vi "Clear Hardware.vi"(2 "error in (no error)":errorcluster, 3 "NI Card in":refnum<class "NI Card.lvclass">) -> (0 "error out":errorcluster, 1 "NI Card out":refnum<class "NI Card.lvclass">)   [LabVIEW 2013, in "NI Card.lvclass"]
uses:
  NI Card.lvclass
  NI Card.lvclass/NI Card.ctl
  <vilib>/DAQmx/read.llb/DAQmx Read (Analog 1D DBL NChan 1Samp).vi
  <vilib>/DAQmx/read.llb/DAQmx Read (Analog 1D Wfm NChan NSamp).vi
  <vilib>/DAQmx/write.llb/DAQmx Write (Analog 1D DBL NChan 1Samp).vi
  <vilib>/DAQmx/miscellaneous.llb/DAQmx Fill In Error Info.vi
  <vilib>/Waveform/WDTOps.llb/WDT Append Waveforms DBL.vi
  <resource>/objmgr/daqmx.rc
panel:
  out "AI Data":cluster{dbl[], "Y":dbl[], "String":string}[](array[cluster])
  out "data":waveform(dbl)[](graph)
  out "First Data Point":dbl[](array[numeric]) format="%0.2f"
  out "Number of points read":i32[](array[numeric])
  in  "Set to zero":bool
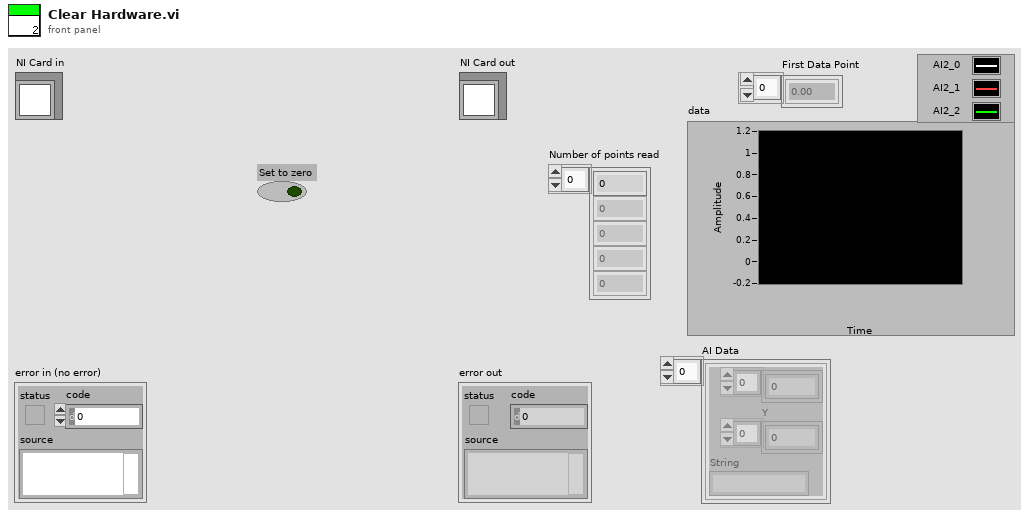
[diagram p1: front panel]
types:
  T1 = cluster{"DAQmx Global Channel":refnum<k21>, "String":string}[]
  T2 = typedef "NI Card.lvclass/AI_Data.ctl" = cluster{"t":dbl[], "y":dbl[], "Channel Name":string}
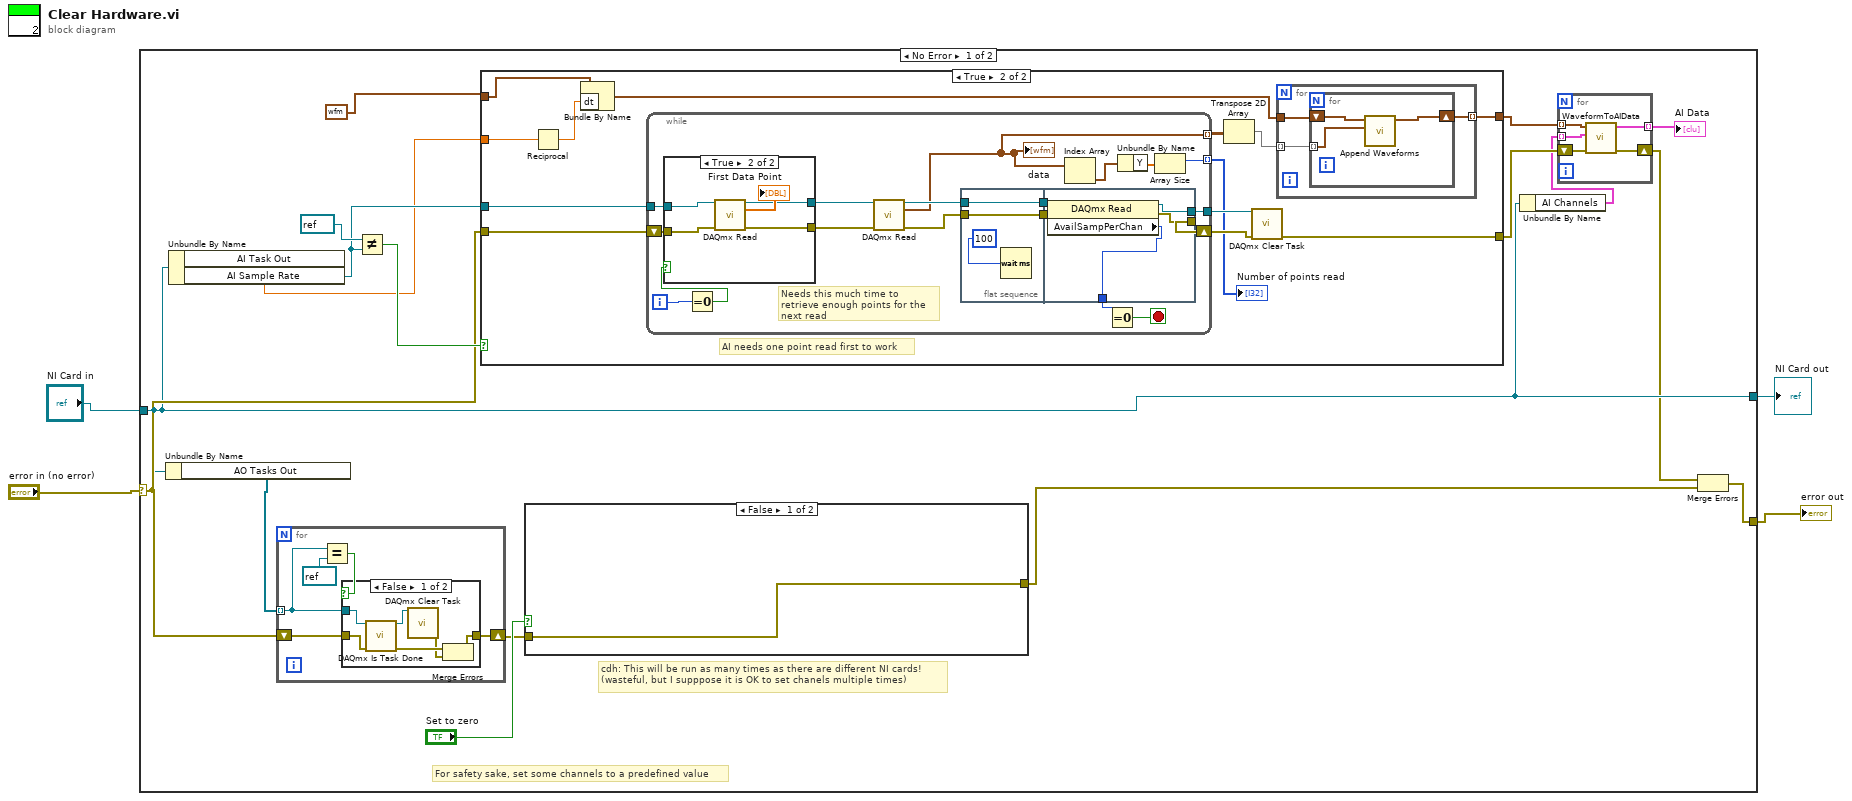
[diagram p0: block diagram]
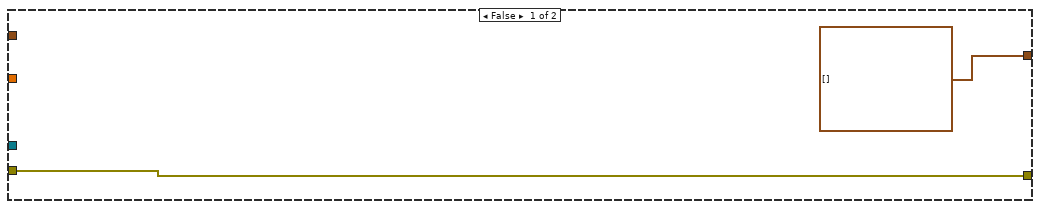
[diagram p2: hidden frame]
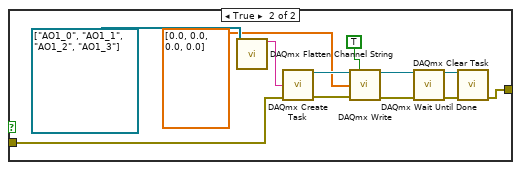
[diagram p5: hidden frame]
diagram:
  n1 = case shown="No Error" "error in (no error)" {
    selector: "error in (no error)" -> [w16 w106]
    tunnel: [w10 w107] -> w1
    tunnel: "NI Card in" -> [w10 w107]
    tunnel: [w6 w106] -> w2
    frame No Error {
      # "cdh: This will be run as many times as there are different NI cards!\n(wasteful, but I supppose it is OK to set chanels multiple times)"
      # "For safety sake, set some channels to a predefined value"
      n2 = Unbundle By Name(w10) -> ("AO Tasks Out"=w21:refnum<k21>[])
      n3 = Unbundle By Name(w10) -> ("AI Task Out"=w15:refnum<k21>, "AI Sample Rate"=w14:dbl)
      n4 = for {
        shift-right: [w82] -> w19
        shift-left: w16 -> [w85]
        tunnel: w21 -> [w81] mode=indexing
        n5 = Equal?(x=w81, y=refnum<k21> refnum ("Name")) -> (x = y?=w83:bool)
        n6 = case shown="False" w83 {
          tunnel: w85 -> [w89 w92]
          tunnel: [w86 w92] -> w82
          tunnel: w81 -> [w91 _]
          frame False {
            n7 = call <vilib>:"DAQmx Is Task Done.vi"("task/channels in"=w91, "error in"=w89) -> ("task out"=w90:refnum<k21>, "error out"=w88:errorcluster)  [unwired: 11 in, 1 out]
            n8 = call <vilib>:"DAQmx Clear Task.vi"("task in"=w90) -> ("error out"=w87:errorcluster)  [unwired: 1 in, 13 out]
            n9 = Merge Errors(w88, w87) -> (w86:errorcluster)
          }
          frame True {
          }
        }
      }
      n10 = Not Equal?(x=refnum<k21> refnum ("task out"), y=w15) -> (x != y?=w17:bool)
      n11 = case shown="True" w17 {
        tunnel: w15 -> [_ w38]
        tunnel: w16 -> [w27 w37]
        tunnel: [w27 w36] -> w11
        tunnel: [waveform(dbl)[] [] w33] -> w12
        tunnel: waveform(dbl) {"t0"=timestamp(0 s since 1904-01-01), "dt"=0.001, "Y"=[]} ("Waveform") -> [_ w31]
        tunnel: w14 -> [_ w29]
        frame False {
        }
        frame True {
          # "AI needs one point read first to work"
          n12 = Reciprocal(x=w29) -> (1/x=w30:dbl)
          n13 = Bundle By Name(cluster=w31, "dt"=w30) -> (w32:waveform(dbl))
          n14 = while {
            tunnel: w38 -> [w64]
            tunnel: [w58] -> w39 mode=indexing
            tunnel: [w54] -> w40
            tunnel: [w48] -> w35 mode=indexing
            shift-right: [w53] -> w41
            shift-left: w37 -> [w63]
            i -> [w51]
            stop <- w57 stop-if-true
            # "Needs this much time to retrieve enough points for the next read"
            n15 = Equal To 0?(x=w51) -> (x = 0?=w50:bool)
            n16 = case shown="True" w50 {
              tunnel: w64 -> [w67 w72]
              tunnel: w63 -> [w66 w71]
              tunnel: [w67 w69] -> w62
              tunnel: [w66 w68] -> w61
              frame False {
              }
              frame True {
                n17 = call-poly <vilib>:"DAQmx Read.vi"("task/channels in"=w72, "error in"=w71) -> ("task out"=w69:refnum<k21>, "data"=→"First Data Point":dbl[], "error out"=w68:errorcluster)  [unwired: 11 out]
              }
            }
            n18 = call-poly <vilib>:"DAQmx Read.vi"("task/channels in"=w62, "error in"=w61) -> ("task out"=w60:refnum<k21>, "data"=w48:waveform(dbl)[], "error out"=w59:errorcluster)  [unwired: 1 in, 10 out]
            "data" <- w48
            n19 = flat-sequence {
              tunnel: w60 -> [w74]
              tunnel: w59 -> [w73]
              tunnel: [w74] -> w56
              tunnel: [w73] -> w55
              tunnel: w56 -> [w80]
              tunnel: w55 -> [w79]
              tunnel: [w78] -> w54
              tunnel: [w77] -> w53
              tunnel: [w76] -> w52
              frame #0 {
                n20 = Wait (ms)(milliseconds to wait=u32 100) -> ()  [unwired: 1 out]
              }
              frame #1 {
                n21 = property class="DAQmx Read"(reference=w80, error in=w79) -> (reference out=w78:refnum<k21>, error out=w77:errorcluster, "AvailSampPerChan"=w76:u32)
              }
            }
            n22 = Index Array(array=w48) -> (element=w49:waveform(dbl))  [unwired: 1 in]
            n23 = Equal To 0?(x=w52) -> (x = 0?=w57:bool)
            n24 = Unbundle By Name(w49) -> ("Y"=w65:dbl[])
            n25 = Array Size(array=w65) -> (size(s)=w58:i32)
          }
          "Number of points read" <- w39
          n26 = Transpose 2D Array(2D array=w35) -> (transposed array=w34:waveform(dbl)[][])
          n27 = call <vilib>:"DAQmx Clear Task.vi"("task in"=w40, "error in"=w41) -> ("error out"=w36:errorcluster)  [unwired: 13 out]
          n28 = for {
            tunnel: w34 -> [w42] mode=indexing
            tunnel: [w43] -> w33 mode=indexing
            tunnel: w32 -> [w44]
            n29 = for {
              tunnel: w42 -> [w45] mode=indexing
              shift-right: [w47] -> w43
              shift-left: w44 -> [w46]
              n30 = call-poly <vilib>:"Append Waveforms.vi"("waveform B"=w45, "waveform A"=w46) -> ("waveform out"=w47:waveform(dbl))  [unwired: 1 in, 8 out]
            }
          }
        }
      }
      n31 = case shown="False" "Set to zero" {
        tunnel: w19 -> [w93 w97]
        tunnel: [w93 w103] -> w7
        frame False {
        }
        frame True {
          n32 = call <vilib>:"DAQmx Flatten Channel String.vi"("names in"=refnum<k21>[] ["AO1_0", "AO1_1", "AO1_2", "AO1_3"]) -> ("names out"=w96:string)  [unwired: 1 in, 13 out]
          n33 = call <vilib>:"DAQmx Create Task.vi"("global virtual channels"=w96, "error in"=w97) -> ("task out"=w102:refnum<k21>, "error out"=w101:errorcluster)  [unwired: 3 in, 9 out]
          n34 = call-poly <vilib>:"DAQmx Write.vi"("task/channels in"=w102, "auto start"=TRUE, "data"=dbl[] [0.0, 0.0, 0.0, 0.0], "error in"=w101) -> ("task out"=w99:refnum<k21>, "error out"=w98:errorcluster)  [unwired: 10 out]
          n35 = call <vilib>:"DAQmx Wait Until Done.vi"("task/channels in"=w99, "error in"=w98) -> ("task out"=w105:refnum<k21>, "error out"=w104:errorcluster)  [unwired: 1 in, 11 out]
          n36 = call <vilib>:"DAQmx Clear Task.vi"("task in"=w105, "error in"=w104) -> ("error out"=w103:errorcluster)  [unwired: 13 out]
        }
      }
      n37 = Unbundle By Name(w10) -> ("AI Channels"=w9:T1)
      n38 = for {
        tunnel: w12 -> [w24] mode=indexing
        tunnel: [w22] -> w5 mode=indexing
        shift-right: [w25] -> w8
        shift-left: w11 -> [w26]
        tunnel: w9 -> [w23] mode=indexing
        n39 = call "WaveformToAIData.vi"("error in (no error)"=w26, "AI Channel"=w23, "AI Waveform"=w24) -> ("error out"=w25:errorcluster, "AI Data"=w22:T2)  [unwired: 7 in]
      }
      "AI Data" <- w5
      n40 = Merge Errors(w8, w7) -> (w6:errorcluster)
    }
    frame Error {
    }
  }
  "error out" <- w2
  "NI Card out" <- w1
